vi "Default Name.vi"() -> (0 "String":string)   [LabVIEW 2009, in "Caraya.lvlib" / "Assert.lvclass"]
uses:
  Assert.lvclass
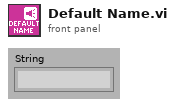
[diagram p1: front panel]
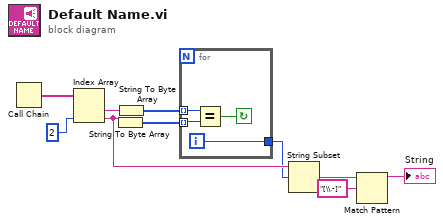
[diagram p0: block diagram]
diagram:
  n1 = Call Chain() -> (call chain=w9:string[])
  n2 = Index Array(array=w9, index #2=2 ("index")) -> (element #1=w8:string, element #2=w5:string)  [unwired: 1 in]
  n3 = String To Byte Array(string=w5) -> (unsigned byte array=w6:u8[])
  n4 = String To Byte Array(string=w8) -> (unsigned byte array=w7:u8[])
  n5 = for {
    tunnel: w7 -> [w14] mode=indexing
    tunnel: w6 -> [w13] mode=indexing
    tunnel: [w11] -> w4
    i -> [w11]
    stop <- w12 continue-if-true
    n6 = Equal?(x=w14, y=w13) -> (x = y?=w12:bool)
  }
  n7 = String Subset(string=w5, offset (0)=w4) -> (substring=w3:string)  [unwired: 1 in]
  n8 = Match Pattern(string=w3, regular expression="[\\.-]") -> (before substring=→"String":string)  [unwired: 1 in, 3 out]
